vi "Handle Last Ack Core.vi"(4 "error in (no error)":errorcluster, 6 "Last Ack":refnum<class "Last Ack.lvclass">, 7 "CI Mediator in":refnum<class "CI Mediator.lvclass">) -> (0 "error out":errorcluster, 3 "CI Mediator out":refnum<class "CI Mediator.lvclass">)   [LabVIEW 2014, in "CI Mediator.lvlib" / "CI Mediator.lvclass"]
doc: "(<B>Filename</B>: Actor Framework.lvlib:Actor.lvclass:Handle Last Ack Core.vi)\n\nDefines how the caller actor responds to the Last Ack message from a nested actor. The Last Ack message is the final message a nested actor sends to its caller before it shuts down. The message contains information about the final state of the nested actor.\n\nBy default, this method does nothing except return any error the nested actor sent. A descendant class may override this method to define behavior."
uses:
  CI Mediator.lvclass
  <vilib>/ActorFramework/LastAck/Last Ack.lvclass
  Jobber Proxy/Jobber Proxy/Jobber Proxy.lvclass
  <vilib>/ActorFramework/LastAck/Last Ack.lvclass/Last Ack.ctl
  Jobber Proxy/Jobber Proxy/Jobber Proxy.lvclass/Jobber Proxy.ctl
  Classes/Job/Job.lvclass/Job.ctl
  CI Mediator.lvclass/CI Mediator.ctl
  <vilib>/ActorFramework/Actor/Actor.lvclass/Actor.ctl
  <vilib>/ActorFramework/Message Enqueuer/Message Enqueuer.lvclass/Message Enqueuer.ctl
  <vilib>/ActorFramework/Message Enqueuer/Init from Existing Queue.vi
  <vilib>/ActorFramework/Message Enqueuer/Enqueue.vi
  <vilib>/ActorFramework/Message Priority Queue/Priority Enqueue.vi
  <vilib>/ActorFramework/Message Enqueuer/Message Enqueuer.lvclass
  <vilib>/ActorFramework/Stop Msg/Stop Msg.lvclass
  <vilib>/ActorFramework/Actor/Actor.lvclass
  Classes/Job/Job.lvclass
  Classes/Executor/Executor.lvclass
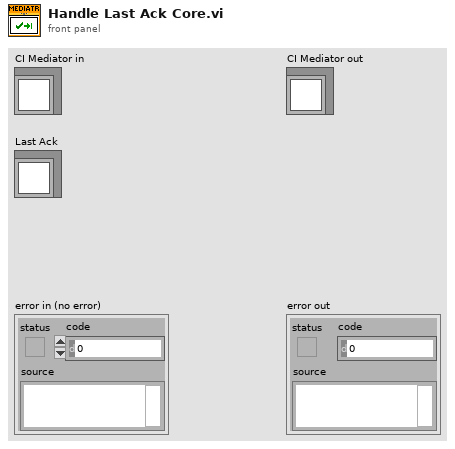
[diagram p1: front panel]
types:
  T1 = typedef "Job Results - STYP.ctl" = cluster{"Status":u16, "Text":string, "Executor Number":i32}
  T2 = typedef "Executor Status - STYP.ctl" = cluster{"Executor Name":string, "Status":bool}
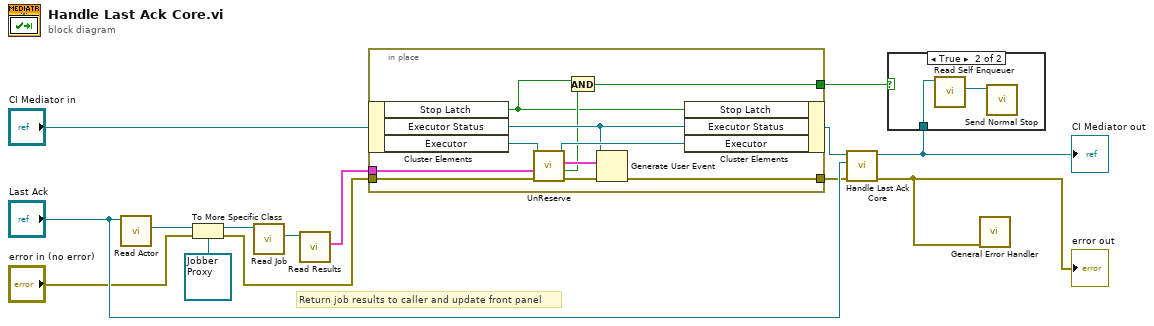
[diagram p0: block diagram]
diagram:
  # "Return job results to caller and update front panel"
  n1 = call <vilib>:"Read Actor.vi"("Last Ack"="Last Ack") -> ("Actor"=w11:refnum<class "Actor.lvclass">)  [unwired: 10 in]
  n2 = To More Specific Class(target class=refnum<class "Jobber Proxy.lvclass"> refnum ("Jobber Proxy.lvlib:Jobber Proxy.lvclass"), reference=w11, error in="error in (no error)") -> (specific class reference=w13:refnum<class "Jobber Proxy.lvclass">, error out=w6:errorcluster)
  n3 = call "Read Job.vi"("Jobber Proxy in"=w13) -> ("Job"=w14:refnum<class "Job.lvclass">)  [unwired: 10 in]
  n4 = call "Read Results.vi"("Job in"=w14) -> ("Results"=w4:T1)  [unwired: 10 in]
  n5 = in-place {
    in-place-border: w6 -> [w23]
    in-place-border: [w20] -> w5
    in-place-border: w4 -> [w21]
    in-place-border: [w15] -> w3
    n6 = in-place-cluster #1("CI Mediator in") -> ("Stop Latch"=w16:bool, "Executor Status"=w18:refnum<user-event>, "Executor"=w25:refnum<class "Executor.lvclass">)
    n7 = call "UnReserve.vi"("error in (no error)"=w23, "Job Results"=w21, "Executor"=w25) -> ("error out"=w22:errorcluster, "Safe Shutdown?"=w17:bool, "Executor States"=w19:T2[], "Executor"=w24:refnum<class "Executor.lvclass">)  [unwired: 5 in]
    n8 = And(x=w16, y=w17) -> (x .and. y?=w15:bool)
    n9 = Generate User Event(user event=w18, event data cluster=w19, error in=w22) -> (error out=w20:errorcluster)  [unwired: 1 in, 1 out]
    n10 = in-place-cluster #1("Stop Latch"=w16, "Executor Status"=w18, "Executor"=w24) -> (w7:refnum<class "CI Mediator.lvclass">)
  }
  n11 = call-parent "Handle Last Ack Core.vi"("error in (no error)"=w5, "Last Ack"="Last Ack", "Actor in"=w7) -> ("error out"=w1:errorcluster, "Actor out"=w2:refnum<class "CI Mediator.lvclass">)  [unwired: 3 in]
  "CI Mediator out" <- w2
  "error out" <- w1
  n12 = case shown="True" w3 {
    tunnel: w2 -> [_ w27]
    frame False {
    }
    frame True {
      n13 = call <vilib>:"Read Self Enqueuer.vi"("Actor"=w27) -> ("Self Enqueuer"=w26:refnum<class "Message Enqueuer.lvclass">)  [unwired: 10 in]
      n14 = call <vilib>:"Send Normal Stop.vi"("Message Enqueuer"=w26) -> ()  [unwired: 10 in, 1 out]
    }
  }
  n15 = call <vilib>:"General Error Handler.vi"("error in (no error)"=w1) -> ()  [unwired: 10 in, 5 out]
